vi "setDAQ.vi"(8 "error in (no error)":errorcluster, 10 "setDAQ":variant, 11 "Instrument.LockinAPI in":refnum<class "Instrument.LockinAPI.lvclass">) -> (0 "error out":errorcluster, 3 "Instrument.LockinAPI out":refnum<class "Instrument.LockinAPI.lvclass">)   [LabVIEW 2019, in "Instrument.LockinAPI.lvclass"]
doc: "API to configure AO.\n\nIf address=\"\", this API reads from localhost\nIf address is remote lockin, you need to add this computer to allowed whitelist on the lockin computer you are trying to access."
uses:
  Instrument.LockinAPI.lvclass
  C:/Users/patrick/Documents/GitHub/Instrument-Framework/lvsrc/Instrument/Instrument.lvclass
  Typedefs/LockinAPI.Commands--Enum.ctl
  8dde282f-c95e-4436-9ad4-90c72b51d4bb.vi
  8dde282f-c95e-4436-9ad4-90c72b51d4bb.vi/aa316dd5-9485-44f7-84e7-0c2f557cd2b1.vi
  8dde282f-c95e-4436-9ad4-90c72b51d4bb.vi/aa316dd5-9485-44f7-84e7-0c2f557cd2b1.vi/d9259a98-530d-4dc3-b2f2-e37b10efeefc.vi
  8dde282f-c95e-4436-9ad4-90c72b51d4bb.vi/aa316dd5-9485-44f7-84e7-0c2f557cd2b1.vi/3ad79273-4db5-40a9-bfee-4994e49cc4b2.vi
  Instrument/Protected/Validate API method.vi
  Instrument/Private/Get RC Connection Status.vi
  Instrument/API/Send and Receive.vi
  <vilib>/Utility/Data Type/Get Type Information.vi
  <vilib>/JDP Science/JSONtext/JSON text to Variant.vi
  <vilib>/JDP Science/JSONtext/LVClass Serializer/JSONtext LVClass Serializer.lvclass
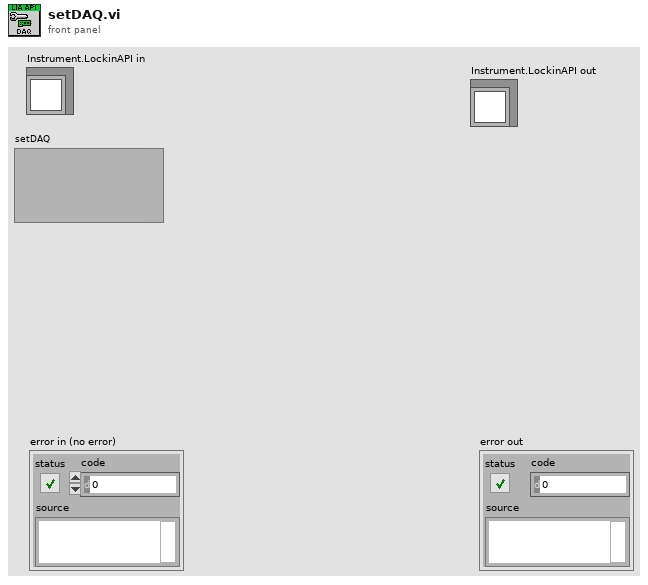
[diagram p1: front panel]
types:
  T1 = typedef "Instrument.LockinAPI.lvclass/LockinAPI.Commands--Enum.ctl" = enum16{"setAI", "setAO", "setAO_Amplitude", "setAO_DC", "setAO_Frequency", "setAO_Phase", "setAO_Function", "setAO_I+", "setREF", "setREF_Frequency", "setREF_Phase", "setREF_TC", "setREF_Roll-Off", "setDAQ", "setSampling", "setOffset", "setState", "getState", "getAO", "getAI", "getResults", "getSampling", "getAOconfig", "getREFconfig", "setInputGain", "setOutputGain", "getInputGain", "getOutputGain", "setSamplingMode", "getSamplingMode", "setSweep", "setSweepTime", "setSweepTable", "getStatus", "getSweepResults", "getSweepWaveforms", "startSweep", "stopSweep", "setAUX", "getAUX"}
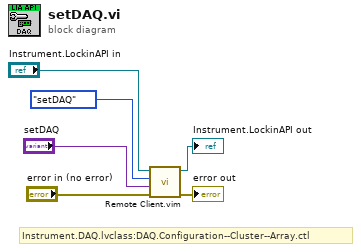
[diagram p0: block diagram]
diagram:
  # "Instrument.DAQ.lvclass:DAQ.Configuration--Cluster--Array.ctl"
  n1 = call "Remote Client.vim"("error in (no error)"="error in (no error)", "Data in"="setDAQ", "Command in"=LockinAPI.Commands--Enum."setDAQ" ("Command"), "Instrument in"="Instrument.LockinAPI in") -> ("error out"=→"error out":errorcluster, "Instrument out"=→"Instrument.LockinAPI out":refnum<class "Instrument.LockinAPI.lvclass">)  [unwired: 4 in, 2 out]
